vi "Add Plugin Thread.vi"(8 "error in (no error)":errorcluster, 9 "priority offset (0)":i16, 10 "processor (-2)":i32=-2, 11 "plugin in":T1={"name"="Plugin", "components"=[], "cycle timing"={"priority"=10000, "decimation"=1, "offset"=0}, "threads"=[], "Transfer Groups"=[], "settings"=[]} {"Transfer Groups"."Transfers"."channels"."string offset" format="%d bytes"}) -> (0 "error out":errorcluster, 2 "plugin thread index":i32, 3 "plugin out":T1={"name"="Plugin", "components"=[], "cycle timing"={"priority"=10000, "decimation"=1, "offset"=0}, "threads"=[], "Transfer Groups"=[], "settings"=[]} {"Transfer Groups"."Transfers"."channels"."string offset" format="%d bytes"})   [LabVIEW 2017, in "DSF Core.lvlib" / "Configuration Session.lvclass"]
doc: "Determines whether a configuration data dsf refnum is valid."
uses:
  Configuration Session.lvclass
  Typedefs/DSF Engine Plugin Configuration.ctl
  Typedefs/DSF Timing Info.ctl
  Typedefs/DSF Engine Plugin Thread Configuration.ctl
  Typedefs/DSF Settings Info.ctl
  Typedefs/DSF Engine Transfer Group Configuration.ctl
  Typedefs/DSF Direction.ctl
  Typedefs/DSF Engine Transfer Configuration.ctl
  Typedefs/DSF Byte Order.ctl
  Typedefs/DSF Engine Channel Configuration.ctl
  Typedefs/DSF Data Type.ctl
  Typedefs/DSF Timeout Behavior.ctl
  DSF Core.lvlib
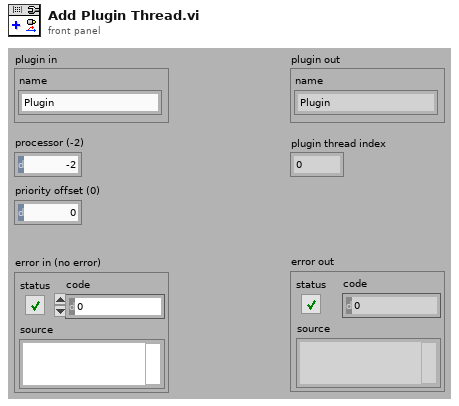
[diagram p1: front panel]
types:
  T1 = typedef "DSF Core.lvlib/DSF Engine Plugin Configuration.ctl" = cluster{"name":string, "components":string[], "cycle timing":T2, "threads":T3[], "Transfer Groups":T5[], "settings":T4}
  T2 = typedef "DSF Core.lvlib/DSF Timing Info.ctl" = cluster{"priority":u64, "decimation":u64, "offset":u64}
  T3 = typedef "DSF Core.lvlib/DSF Engine Plugin Thread Configuration.ctl" = cluster{"buffer converter settings":T4, "transceiver settings":T4, "custom settings":T4, "processor":i32, "priority offset":i16}
  T4 = typedef "DSF Core.lvlib/DSF Settings Info.ctl" = cluster{"key":string, "value":string}[]
  T5 = typedef "DSF Core.lvlib/DSF Engine Transfer Group Configuration.ctl" = cluster{"name":string, "direction":T6, "cycle timing":T2, "thread index":i32, "settings":T4, "Transfers":T7[], "timeout behavior":T11}
  T6 = typedef "DSF Core.lvlib/DSF Direction.ctl" = enum8{"Tx", "Rx"}
  T7 = typedef "DSF Core.lvlib/DSF Engine Transfer Configuration.ctl" = cluster{"name":string, "byte order":T8, "settings":T4, "channels":T9[]}
  T8 = typedef "DSF Core.lvlib/DSF Byte Order.ctl" = enum8{"big-endian", "little-endian"}
  T9 = typedef "DSF Core.lvlib/DSF Engine Channel Configuration.ctl" = cluster{"string offset":u64, "string data type":T10, "engine data type":T10, "name":string, "settings":T4, "units":string}
  T10 = typedef "DSF Core.lvlib/DSF Data Type.ctl" = enum8{"Bool", "SGL", "DBL", "I8", "I16", "I32", "I64", "U8", "U16", "U32", "U64"}
  T11 = typedef "DSF Core.lvlib/DSF Timeout Behavior.ctl" = enum8{"Increment Late Count", "Throw Error"}
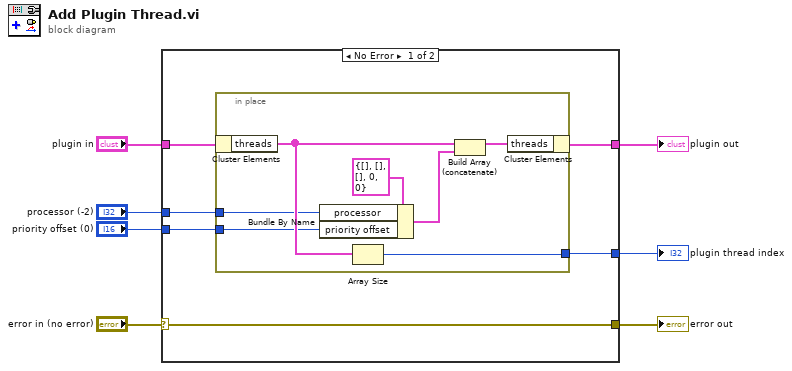
[diagram p0: block diagram]
diagram:
  n1 = case shown="No Error" "error in (no error)" {
    selector: "error in (no error)" -> [w8 w22]
    tunnel: [w8 w22] -> w7
    tunnel: "processor (-2)" -> [w13 _]
    tunnel: "priority offset (0)" -> [w12 _]
    tunnel: [w11 _] -> w3
    tunnel: "plugin in" -> [w10 w21]
    tunnel: [w9 w21] -> w1
    frame No Error {
      n2 = in-place {
        in-place-border: w13 -> [w15]
        in-place-border: w12 -> [w14]
        in-place-border: [w17] -> w11
        n3 = in-place-cluster #1(w10) -> ("threads"=w16:T3[])
        n4 = Bundle By Name(cluster=T3 {"buffer converter settings"=[], "transceiver settings"=[], "custom settings"=[], "processor"=0, "priority offset"=0} ("Plugin Thread Configuration"), "processor"=w15, "priority offset"=w14) -> (w18:T3)
        n5 = Array Size(array=w16) -> (size(s)=w17:i32)
        n6 = Build Array (concatenate)(w16, w18) -> (w20:T3[])
        n7 = in-place-cluster #1("threads"=w20) -> (w9:T1)
      }
    }
    frame Error {
    }
  }
  "error out" <- w7
  "plugin thread index" <- w3
  "plugin out" <- w1
